vi "MFC Test RT.vi"() -> ()   [LabVIEW 2014]
uses:
  <vilib>/FPGAPlugInAG/cRIO-9067/niLvFpga_Open_cRIO-9067.vi
  <vilib>/Utility/error.llb/Error Cluster From Error Code.vi
  <vilib>/rvi/errors/niLvFpgaAdjustHostInterfaceError.vi
  <vilib>/FPGAPlugInAG/cRIO-9067/niLvFpga_Close_cRIO-9067.vi
  <vilib>/rvi/interface/nirviOpenFPGA/nirviOpenFPGA.xnode
  FPGA Bitfiles/MAXCAT_FPGATarget5_MFC10Hz_G8opJjVEjRo.lvbitx
  <vilib>/rvi/interface/nirviReadWriteControl/nirviReadWriteControl.xnode
  <vilib>/rvi/interface/nirviCloseFPGA/nirviCloseFPGA.xnode
  NiFpgaLv.dll
panel:
  in  "Count(mSec)":u32
  out "In Array 2":fxp<+/-,24,9>[](array[numeric])
  out "M7P4 string":string
  out "MFC M7P4":u8[](array[numeric])
  out "MFC M7P4 string":string
  in  "Out Array":u8[](array[numeric])=[66, 48, 48, 48, 48, 48, 13, 67, 48, 48, 48, 48, 48, 13, 73, 48, 48, 48, 48, 48, 13, 74, 48, 48, 48, 48, 48, 13, 75, 48, 48, 48, 48, 48, 13, 0, 0, 0, 0, 0, 0, 0, 0, 0, 0, 0, 0, 0, 0, 0, 0, 0, 0, 0, 0, 0]
  out "MFC M8P1 string":string
  out "M8P1 string":string
  out "MFC M8P1":u8[](array[numeric])
  in  "stop":bool
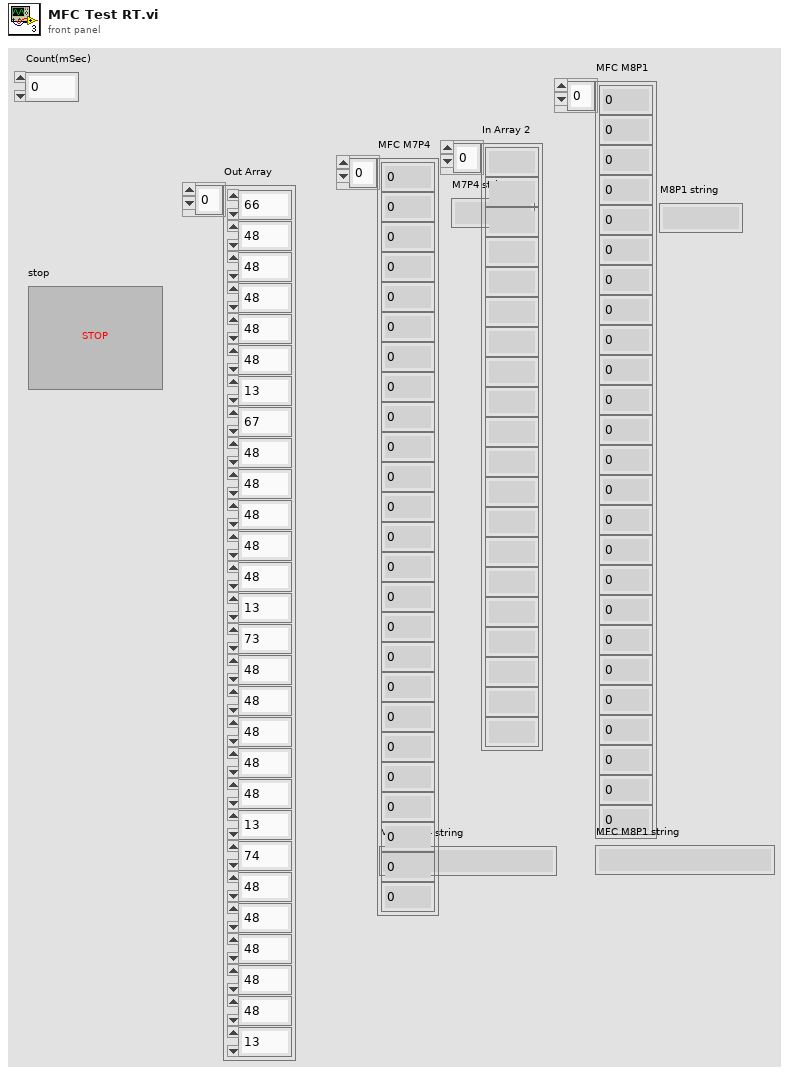
[diagram p1: front panel]
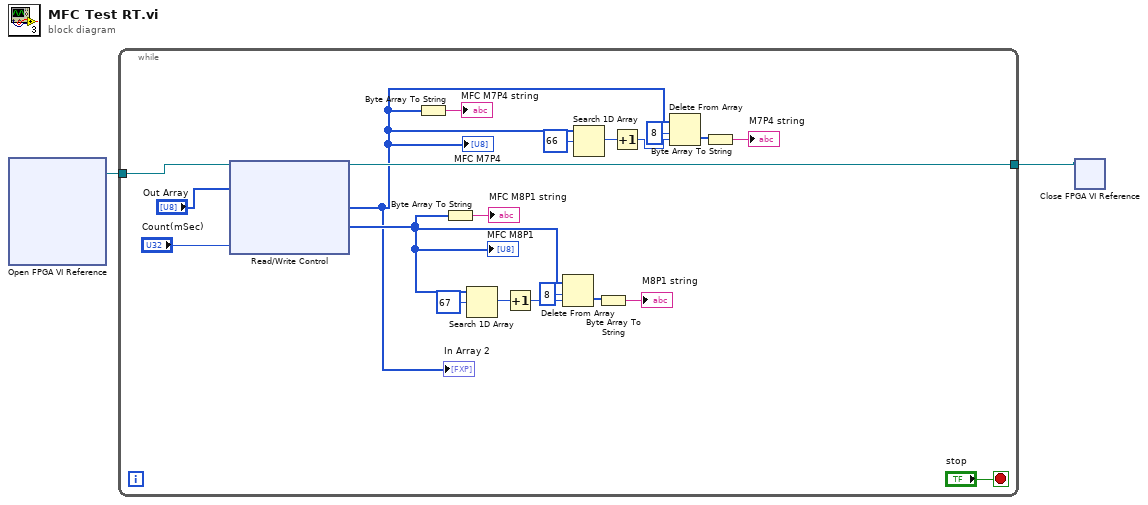
[diagram p0: block diagram]
diagram:
  n1 = xnode "Open FPGA VI Reference"() -> ("FPGA VI Reference Out"=w2:refnum<k20>)  [unwired: 2 in, 1 out]
  n2 = while {
    tunnel: w2 -> [w23]
    tunnel: [w22] -> w1
    stop <- "stop" stop-if-true
    n3 = xnode ("Read/Write Control")("FPGA VI Reference In"=w23, "MFC OUT Array"="Out Array", "Count(mSec)"="Count(mSec)") -> ("FPGA VI Reference Out"=w22:refnum<k20>, "MFC IN Array"=w4:u8[], "MFC AIR-1 out"=w5:u8[])  [unwired: 1 in, 1 out]
    "MFC M8P1" <- w5
    "MFC M7P4" <- w4
    "In Array 2" <- w4
    n4 = Byte Array To String(unsigned byte array=w4) -> (string=→"MFC M7P4 string":string)
    n5 = Byte Array To String(unsigned byte array=w5) -> (string=→"MFC M8P1 string":string)
    n6 = Search 1D Array(1D array=w5, element=u8 67) -> (index of element=w18:i32)  [unwired: 1 in]
    n7 = Increment(x=w18) -> (x+1=w17:i32)
    n8 = Delete From Array(array=w5, length=8, index=w17) -> (deleted portion=w16:u8[])  [unwired: 1 out]
    n9 = Search 1D Array(1D array=w4, element=u8 66) -> (index of element=w8:i32)  [unwired: 1 in]
    n10 = Byte Array To String(unsigned byte array=w16) -> (string=→"M8P1 string":string)
    n11 = Increment(x=w8) -> (x+1=w9:i32)
    n12 = Delete From Array(array=w4, length=8, index=w9) -> (deleted portion=w10:u8[])  [unwired: 1 out]
    n13 = Byte Array To String(unsigned byte array=w10) -> (string=→"M7P4 string":string)
  }
  n14 = xnode "Close FPGA VI Reference"("FPGA VI Reference In"=w1) -> ()  [unwired: 1 in, 1 out]
